vi "SftpListDirectory.vi"(0 "error in":errorcluster, 7 "Robot Path":string, 11 "Sftp":refnum<k24>) -> (4 "error out":errorcluster, 15 "DirectoryItems":T1(array[cluster]))   [LabVIEW 2016, in "UnderAutomation.UniversalRobots.lvlib"]
uses:
  UnderAutomation.UniversalRobots.lvlib
  C:/Users/fg/Documents/UniversalRobots.vi/LabVIEW_2024/UnderAutomation.UniversalRobots/lib/UnderAutomation.UniversalRobots.dll
  LabVIEW_2024/UnderAutomation.UniversalRobots/lib/UnderAutomation.UniversalRobots.dll
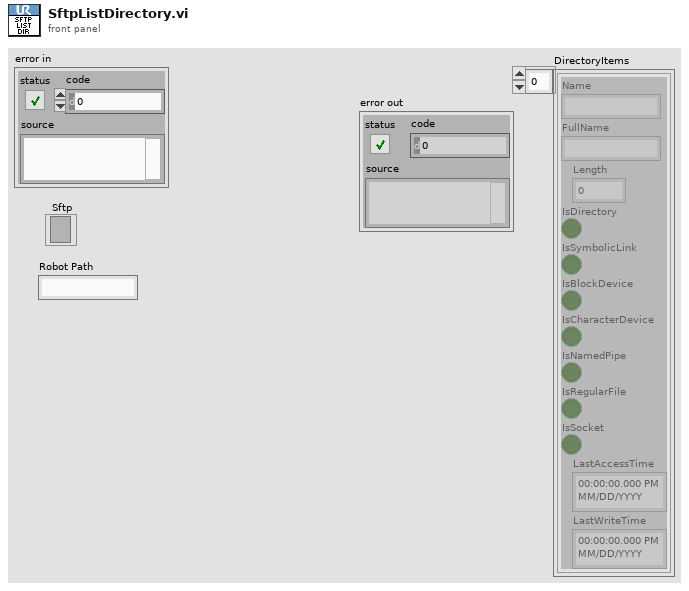
[diagram p1: front panel]
types:
  T1 = cluster{"Name":string, "FullName":string, "Length":i64, "IsDirectory":bool, "IsSymbolicLink":bool, "IsBlockDevice":bool, "IsCharacterDevice":bool, "IsNamedPipe":bool, "IsRegularFile":bool, "IsSocket":bool, "LastAccessTime":timestamp, "LastWriteTime":timestamp}[]
  T2 = cluster{"Name":string, "FullName":string, "Length":i64, "IsDirectory":bool, "IsSymbolicLink":bool, "IsBlockDevice":bool, "IsCharacterDevice":bool, "IsNamedPipe":bool, "IsRegularFile":bool, "IsSocket":bool, "LastAccessTime":timestamp, "LastWriteTime":timestamp}
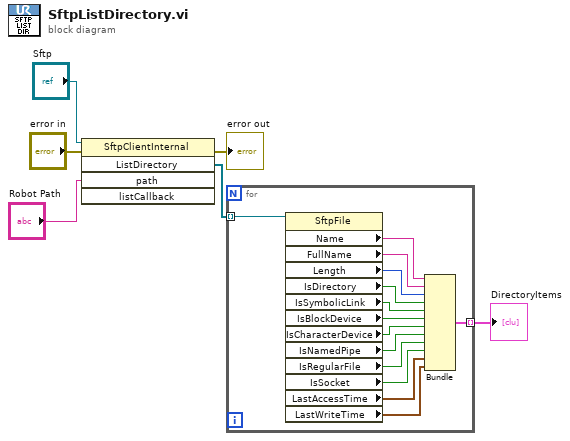
[diagram p0: block diagram]
diagram:
  n1 = invoke class="SftpClientInternal" method="ListDirectory"(reference="Sftp", error in="error in", "path"="Robot Path") -> (error out=→"error out":errorcluster, "ListDirectory"=w2:refnum<k24>[])  [unwired: 2 in, 3 out]
  n2 = for {
    tunnel: w2 -> [w20] mode=indexing
    tunnel: [w17] -> w1 mode=indexing
    n3 = property class="SftpFile"(reference=w20) -> ("Name"=w19:string, "FullName"=w18:string, "Length"=w16:i64, "IsDirectory"=w15:bool, "IsSymbolicLink"=w14:bool, "IsBlockDevice"=w13:bool, "IsCharacterDevice"=w12:bool, "IsNamedPipe"=w11:bool, "IsRegularFile"=w10:bool, "IsSocket"=w9:bool, "LastAccessTime"=w8:timestamp, "LastWriteTime"=w7:timestamp)  [unwired: 1 in, 2 out]
    n4 = Bundle("Name"=w19, "FullName"=w18, "Length"=w16, "IsDirectory"=w15, "IsSymbolicLink"=w14, "IsBlockDevice"=w13, "IsCharacterDevice"=w12, "IsNamedPipe"=w11, "IsRegularFile"=w10, "IsSocket"=w9, "LastAccessTime"=w8, "LastWriteTime"=w7) -> (w17:T2)  [unwired: 1 in]
  }
  "DirectoryItems" <- w1
